vi "test parse tcp replies efficiency.vi"() -> ()   [LabVIEW 2013]
panel:
  out "x = y?":bool[][](array[boolean])
  in  "Array 2":string[][](array[string])=array2x22800[45600 elements]
  out "Array":string[][](array[string])
  out "OK?":bool
  in  "replies":string[](array[string])=["71146 LEPS Interface>>0>>Device Status nval,Initialized nvar,\r\ndevice error nval, nvar,\r\ndevice preset nval, nvar,\r\n", "Avocent-PSU-upstream>>0>>Device Status nval,Initialized nvar,\r\ndevice error nval, nvar,\r\ndevice preset nval, nvar,\r\n", "BellaESP>>0>>Device Status nval,Initialized nvar,\r\ndevice error nval, nvar,\r\ndevice preset nval, nvar,\r\n", "BellaSRS>>0>>Device Status nval,no scan nvar,\r\ndevice error nval, nvar,\r\ndevice preset nval, nvar,\r\n", "BellaSRS2>>0>>Device Status nval,no scan nvar,\r\ndevice error nval, nvar,\r\ndevice preset nval, nvar,\r\n", "BellaTHALESsveECS>>0>>Device Status nval,no scan nvar,\r\ndevice error nval, nvar,\r\ndevice preset nval, nvar,\r\n", "BELLA_ESP_2>>0>>Device Status nval,Initialized nvar,\r\ndevice error nval, nvar,\r\ndevice preset nval, nvar,\r\n", "BELLA_ESP_M1>>0>>Device Status nval,Initialized nvar,\r\ndevice error nval, nvar,\r\ndevice preset nval, nvar,\r\n", "BELLA_filter_wheels>>0>>Device Status nval,Initialized nvar,\r\ndevice error nval, nvar,\r\ndevice preset nval, nvar,\r\n", "BELLA_HallProbe>>0>>Device Status nval,no scan nvar,\r\ndevice error nval, nvar,\r\ndevice preset nval, nvar,\r\n", "BELLA_PDR2000>>0>>Device Status nval,Initialized nvar,\r\ndevice error nval, nvar,\r\ndevice preset nval, nvar,\r\n", "Comp1>>0>>Device Status nval,no scan nvar,\r\ndevice error nval, nvar,\r\ndevice preset nval, nvar,\r\n", "FireContinues>>0>>Device Status nval,no scan nvar,\r\ndevice error nval, nvar,\r\ndevice preset nval, nvar,\r\n", "HamamatsuDAQ>>0>>Device Status nval,no scan nvar,\r\ndevice error nval, nvar,\r\ndevice preset nval, nvar,\r\n", "HASOCopyAA>>0>>Device Status nval,no scan nvar,\r\ndevice error nval,6/7/2018 10:47 AM,1430,Move in FileCopy.lvclass:Save.vi->Device_control.vi<APPEND>\n<Not A Path>\n6/7/2018 10:47 AM,1430,Move in FileCopy.lvclass:Save.vi->Device_control.vi<APPEND>\n<Not A Path>\n\n6/7/2018 10:47 AM,1430,Move in FileCopy.lvclass:Save.vi->Device_control.vi<APPEND>\n<Not A Path>\n\n6/7/2018 10:47 AM,1430,Move in FileCopy.lvclass:Save.vi->Device_control.vi<APPEND>\n<Not A Path> nvar,\r\ndevice preset nval, nvar,\r\n", "HeatESP>>0>>Device Status nval,Initialized nvar,\r\ndevice error nval, nvar,\r\ndevice preset nval, nvar,\r\n", "HeatFF>>0>>Device Status nval,no scan nvar,\r\ndevice error nval, nvar,\r\ndevice preset nval, nvar,\r\n", "HeatFilterwheels>>0>>Device Status nval,Initialized nvar,\r\ndevice error nval, nvar,\r\ndevice preset nval, nvar,\r\n", "HeatHighlandT564>>0>>Device Status nval,no scan nvar,\r\ndevice error nval, nvar,\r\ndevice preset nval, nvar,\r\n", "HeatHPDCCD>>0>>Device Status nval,no scan nvar,\r\ndevice error nval, nvar,\r\ndevice preset nval, nvar,\r\n", "HeatM3HPD>>0>>Device Status nval,no scan nvar,\r\ndevice error nval, nvar,\r\ndevice preset nval, nvar,\r\n", "HeatNF2>>0>>Device Status nval,no scan nvar,\r\ndevice error nval, nvar,\r\ndevice preset nval, nvar,\r\n", "HPD-Far-Stage>>0>>Device Status nval,Initialized nvar,\r\ndevice error nval, nvar,\r\ndevice preset nval, nvar,\r\n", "HPDccd2>>0>>Device Status nval,no scan nvar,\r\ndevice error nval, nvar,\r\ndevice preset nval, nvar,\r\n", "HPDCCD3>>0>>Device Status nval,no scan nvar,\r\ndevice error nval, nvar,\r\ndevice preset nval, nvar,\r\n", "HPDTelescopeStage>>0>>Device Status nval,Initialized nvar,\r\ndevice error nval, nvar,\r\ndevice preset nval, nvar,\r\n", "HPD_CCD>>0>>Device Status nval,no scan nvar,\r\ndevice error nval, nvar,\r\ndevice preset nval, nvar,\r\n", "HPD_EnergyMeter>>0>>Device Status nval,no scan nvar,\r\ndevice error nval, nvar,\r\ndevice preset nval, nvar,\r\n", "LB-Heat_DG535>>0>>Device Status nval,no scan nvar,\r\ndevice error nval, nvar,\r\ndevice preset nval, nvar,\r\n", "LB-Pico-Booster>>0>>Device Status nval,Initialized nvar,\r\ndevice error nval, nvar,\r\ndevice preset nval, nvar,\r\n", "LB-PL-Doubler-TC>>0>>Device Status nval,Initialized nvar,\r\ndevice error nval, nvar,\r\ndevice preset nval, nvar,\r\n", "LB-PL-EnergyMeter>>0>>Device Status nval,no scan nvar,\r\ndevice error nval, nvar,\r\ndevice preset nval, nvar,\r\n", "LB-Tel4TC>>0>>Device Status nval,Initialized nvar,\r\ndevice error nval, nvar,\r\ndevice preset nval, nvar,\r\n", "LB_EnergyMeter_1>>0>>Device Status nval,no scan nvar,\r\ndevice error nval, nvar,\r\ndevice preset nval, nvar,\r\n", "LB_EnergyMeter_2>>0>>Device Status nval,no scan nvar,\r\ndevice error nval, nvar,\r\ndevice preset nval, nvar,\r\n", "LeCroy64Xi>>0>>Device Status nval,no scan nvar,\r\ndevice error nval, nvar,\r\ndevice preset nval, nvar,\r\n", "LT-FW-DM>>0>>Device Status nval,Initialized nvar,\r\ndevice error nval, nvar,\r\ndevice preset nval, nvar,\r\n", "M1Cam>>0>>Device Status nval,no scan nvar,\r\ndevice error nval, nvar,\r\ndevice preset nval, nvar,\r\n", "M3HPD_CCD_Near>>0>>Device Status nval,no scan nvar,\r\ndevice error nval, nvar,\r\ndevice preset nval, nvar,\r\n", "ManualFilters1>>0>>Device Status nval,no scan nvar,\r\ndevice error nval, nvar,\r\ndevice preset nval, nvar,\r\n", "Offsets-Timing>>0>>Device Status nval,Initialized nvar,\r\ndevice error nval, nvar,\r\ndevice preset nval, nvar,\r\n", "PL1-FilterWheels>>0>>Device Status nval,Initialized nvar,\r\ndevice error nval, nvar,\r\ndevice preset nval, nvar,\r\n", "PL1-GlassmanHV>>0>>Device Status nval,no scan nvar,\r\ndevice error nval, nvar,\r\ndevice preset nval, nvar,\r\n", "PL1-Hexapod>>0>>Device Status nval,Initialized nvar,\r\ndevice error nval, nvar,\r\ndevice preset nval, nvar,\r\n", "PL1-PresCtrl-Low1>>0>>Device Status nval,Initialized nvar,\r\ndevice error nval, nvar,\r\ndevice preset nval, nvar,\r\n", "PL1-PresCtrl-Low2>>0>>Device Status nval,Initialized nvar,\r\ndevice error nval, nvar,\r\ndevice preset nval, nvar,\r\n", "PL1-SideSpec>>0>>Device Status nval,no scan nvar,\r\ndevice error nval, nvar,\r\ndevice preset nval, nvar,\r\n", "PL1-SideView>>0>>Device Status nval,no scan nvar,\r\ndevice error nval, nvar,\r\ndevice preset nval, nvar,\r\n", "PL1-Stage-Cap>>0>>Device Status nval,no scan nvar,\r\ndevice error nval, nvar,\r\ndevice preset nval, nvar,\r\n", "Qred>>0>>Device Status nval,no scan nvar,\r\ndevice error nval, nvar,\r\ndevice preset nval, nvar,\r\n", "RegenSpectrometer>>0>>Device Status nval,no scan nvar,\r\ndevice error nval, nvar,\r\ndevice preset nval, nvar,\r\n", "SmaractFilter-1>>0>>Device Status nval,no scan nvar,\r\ndevice error nval, nvar,\r\ndevice preset nval, nvar,\r\n", "SRS0>>0>>Device Status nval,Initialized nvar,\r\ndevice error nval, nvar,\r\ndevice preset nval, nvar,\r\n", "Targets_HeatHPDCCD>>0>>Device Status nval,Initialized nvar,\r\ndevice error nval, nvar,\r\ndevice preset nval, nvar,\r\n", "Targets_HPDccd2>>0>>Device Status nval,Initialized nvar,\r\ndevice error nval, nvar,\r\ndevice preset nval, nvar,\r\n", "Targets_HPD_CCD>>0>>Device Status nval,Initialized nvar,\r\ndevice error nval, nvar,\r\ndevice preset nval, nvar,\r\n", "XtalLogging>>0>>Device Status nval,Initialized nvar,\r\ndevice error nval, nvar,\r\ndevice preset nval, nvar,\r\n"]
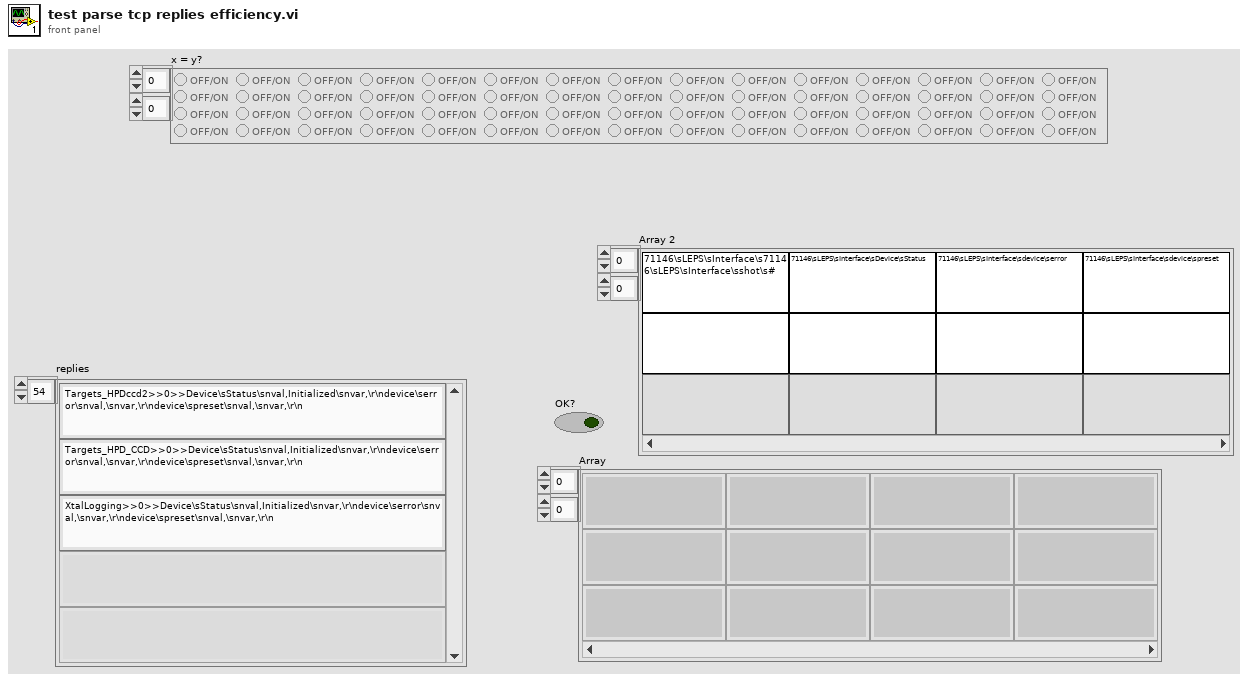
[diagram p1: front panel]
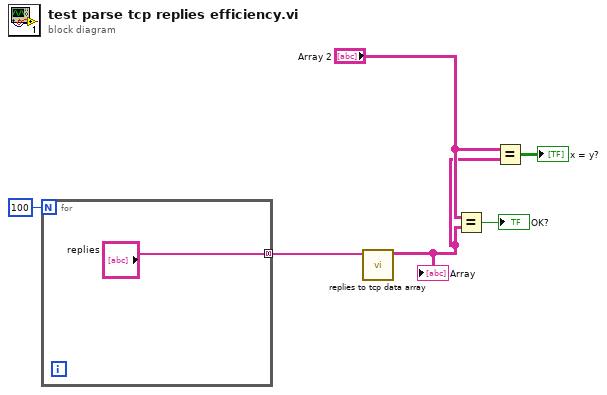
[diagram p0: block diagram]
diagram:
  n1 = for {
    N: 100 -> [_]
    tunnel: ["replies"] -> w6 mode=concatenating
  }
  n2 = call "replies to tcp data array.vi"("replies"=w6) -> ("Array"=w2:string[][])  [unwired: 9 in, 1 out]
  "Array" <- w2
  n3 = Equal?(x="Array 2", y=w2) -> (x = y?=→"OK?":bool)
  n4 = Equal?(x="Array 2", y=w2) -> (x = y?=→"x = y?":bool[][])
